vi "write_pulse_1_ch per device.vi"(8 "error in (no error)":errorcluster, 9 "type":u64, 10 "Array tdms":refnum<k34>[](array[refnum]), 11 "fpga_":refnum<k20>[](array[refnum])) -> (0 "error in (no error) 2":errorcluster, 1 "num of pulse sent to fpga":i32, 2 "done write file":bool[](array[boolean]), 3 "tdms":refnum<k34>[](array[refnum]))   [LabVIEW 2022 SP3]
uses:
  <vilib>/Utility/error.llb/Error Cluster From Error Code.vi
  <vilib>/rvi/errors/niLvFpgaAdjustHostInterfaceError.vi
  <vilib>/rvi/interface/nirviMethod/nirviMethod.xnode
  <vilib>/FPGAPlugInAG/Dynamic/niLvFpga_WriteFifo_Dynamic.vi
  <vilib>/rvi/errors/niLvFpgaMergeErrorWithErrorCode.vi
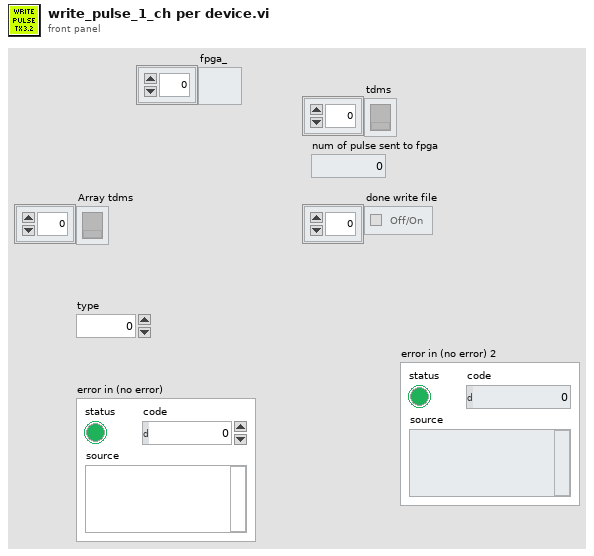
[diagram p1: front panel]
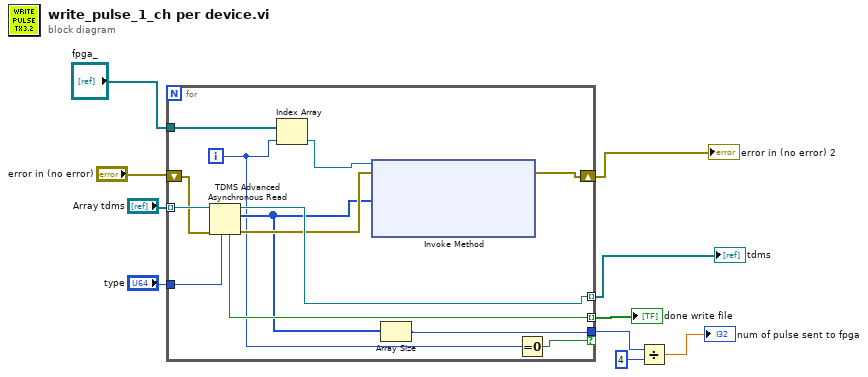
[diagram p0: block diagram]
diagram:
  n1 = for {
    tunnel: "Array tdms" -> [w23] mode=indexing
    tunnel: "fpga_" -> [w22]
    tunnel: "type" -> [w20]
    tunnel: [w19] -> w9 mode=indexing
    tunnel: [w18] -> w10 mode=indexing
    shift-right: [w16] -> w5
    shift-left: "error in (no error)" -> [w15]
    tunnel: [w13] -> w4 if=w12
    i -> [w11]
    n2 = TDMS Advanced Asynchronous Read(6:w20, 8:w15, 11:w23) -> (0:w17:errorcluster, 2:w14:u64[], 3:w18:refnum<k34>, 4:w19:bool)
    n3 = Index Array(array=w22, index=w11) -> (element=w21:refnum<k20>)
    n4 = xnode "Invoke Method"("FPGA VI Reference In"=w21, "error in"=w17, "Data"=w14) -> ("error out"=w16:errorcluster)  [unwired: 1 in, 2 out]
    n5 = Array Size(array=w14) -> (size(s)=w13:i32)
    n6 = Equal To 0?(x=w11) -> (x = 0?=w12:bool)
  }
  "tdms" <- w10
  "done write file" <- w9
  "error in (no error) 2" <- w5
  n7 = Divide(x=w4, y=4) -> (x/y=→"num of pulse sent to fpga":dbl)
